vi "Create.vi"(0 "Test Log Factory in":refnum<class "Test Log Factory.lvclass">, 5 "Test Log Types":T1, 7 "Test Name":string, 9 "Scan Name":string, 11 "error in (no error)":errorcluster) -> (4 "Test Log Factory out":refnum<class "Test Log Factory.lvclass">, 6 "Test Log":refnum<class "Test Log.lvclass">, 15 "error out":errorcluster)   [LabVIEW 2016, in "Test Log Factory.lvclass"]
uses:
  Test Log Factory.lvclass
  Test Log/Test Log.lvclass
  Typedefs/TestLogTypes.ctl
  CSV Test Log/CSV Test Log.lvclass
  C:/CODE/ts_hpmt/Model/Test Log/Test Log/Test Log.lvclass
  Typedefs/LogPath.ctl
  Typedefs/HPMT_Typedefs.lvlib
  Settings/Settings.lvclass
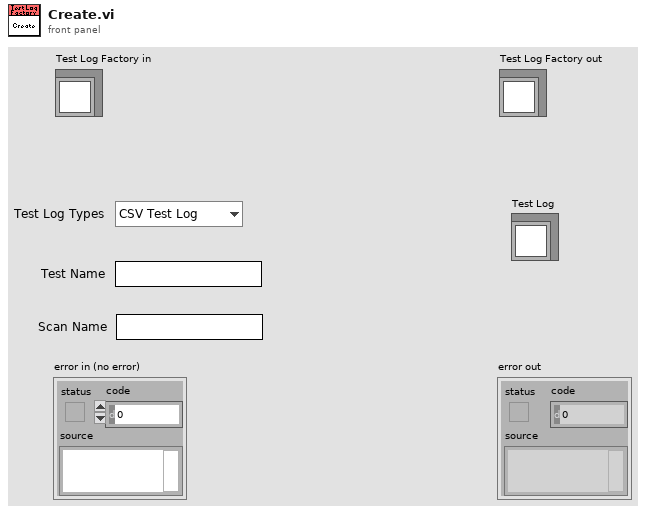
[diagram p1: front panel]
types:
  T1 = typedef "HPMT_Typedefs.lvlib/TestLogTypes.ctl" = enum16{"CSV Test Log"}
  T2 = typedef "HPMT_Typedefs.lvlib/LogPath.ctl" = path
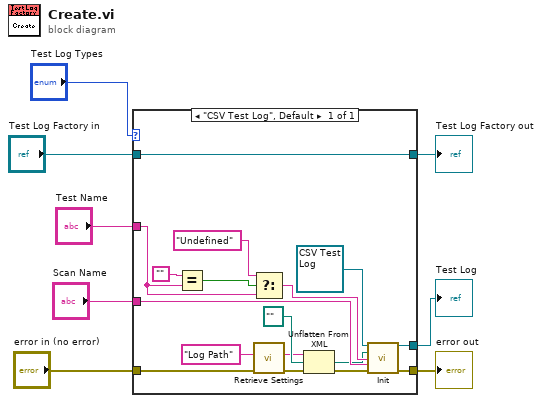
[diagram p0: block diagram]
diagram:
  n1 = case shown="\"CSV Test Log\", Default" "Test Log Types" {
    tunnel: "error in (no error)" -> [w11]
    tunnel: [w24] -> w3
    tunnel: [w20] -> w4
    tunnel: [w25] -> w2
    tunnel: "Test Log Factory in" -> [w25]
    tunnel: "Test Name" -> [w17]
    tunnel: "Scan Name" -> [w14]
    frame "CSV Test Log", Default {
      n2 = Equal?(x="", y=w17) -> (x = y?=w18:bool)
      n3 = Select(t="Undefined", s=w18, f=w17) -> (s? t:f=w16:string)
      n4 = call "Retrieve Settings.vi"("error in (no error)"=w11, "configName"="Log Path") -> ("error out"=w10:errorcluster, "xmlConfig"=w9:string)  [unwired: 7 in, 1 out]
      n5 = Unflatten From XML(xml string=w9, type=T2 path "" ("Log Path"), error in (no error)=w10) -> (value=w13:T2, error out=w21:errorcluster)
      n6 = call "Init.vi"("CSV Test Log in"=refnum<class "CSV Test Log.lvclass"> refnum ("CSVTestLog.lvclass"), "Log Path"=w13, "Test Name"=w16, "Scan Name"=w14, "error in (no error)"=w21) -> ("CSV Test Log out"=w24:refnum<class "CSV Test Log.lvclass">, "error out"=w20:errorcluster)  [unwired: 9 in]
    }
  }
  "error out" <- w4
  "Test Log Factory out" <- w2
  "Test Log" <- w3
